vi "Menu Button Facade.vi"(0 "Data In":T4, 2 "Display State In":T2, 3 "Container State":T3) -> (6 "Data Out":T4, 7 "Display State Out":T2, 8 "Action":T1)   [LabVIEW 2011, in "Menu Button Library.lvlib" / "Menu Button xControl.xctl"]
uses:
  Menu Button xControl.xctl
  Menu Button Data.ctl
  <vilib>/_xctls/Container State.ctl
  Menu Button State.ctl
  <vilib>/_xctls/Action.ctl
  <vilib>/_xctls/XControlSupport.lvlib
panel:
  out "Button 0":string
types:
  T1 = typedef "XControlSupport.lvlib/Action.ctl" = cluster{"Data Changed?":bool, "State Changed?":bool, "Action Name":string}
  T2 = typedef "Menu Button Library.lvlib/Menu Button xControl.xctl/Menu Button State.ctl" = cluster{"Number":i32, "Button Text":string, "Background Color":u32}
  T3 = typedef "XControlSupport.lvlib/Container State.ctl" = cluster{"Indicator?":bool, "Run Mode?":bool, " Refnum":refnum<vi>}
  T4 = typedef "Menu Button Library.lvlib/Menu Button xControl.xctl/Menu Button Data.ctl" = bool
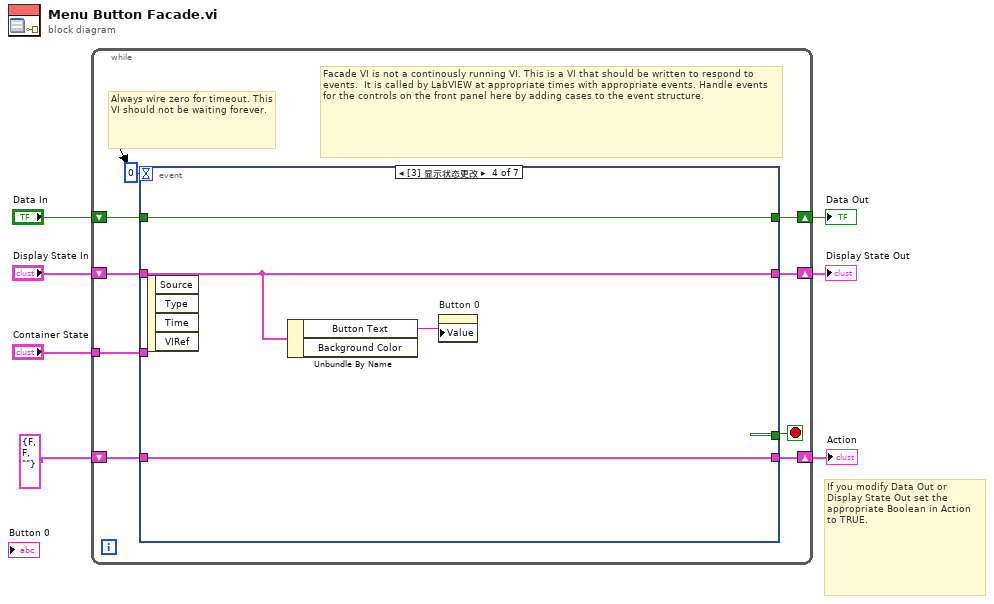
[diagram p0: block diagram]
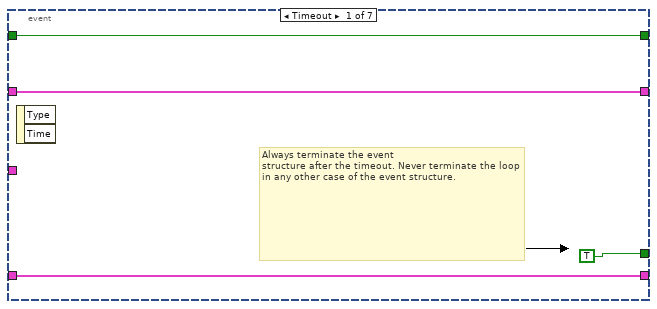
[diagram p2: hidden frame]
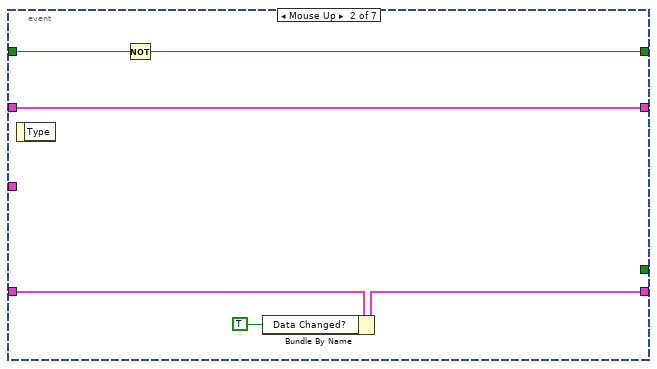
[diagram p3: hidden frame]
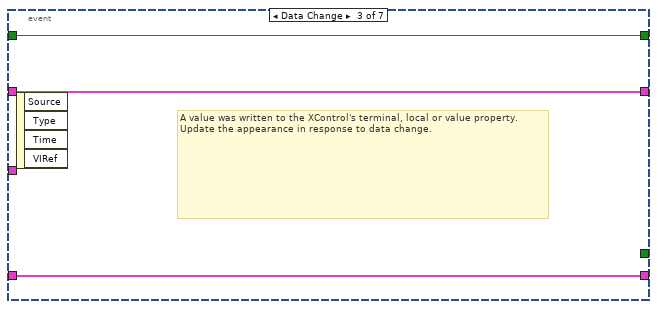
[diagram p4: hidden frame]
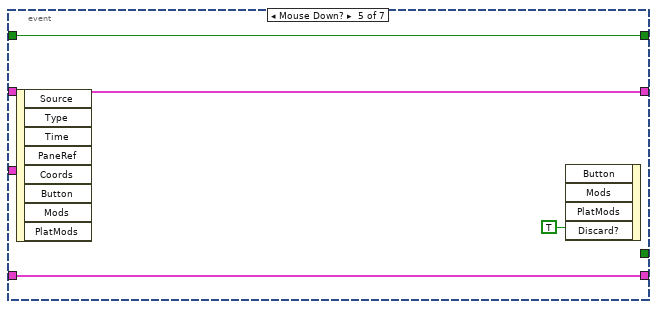
[diagram p5: hidden frame]
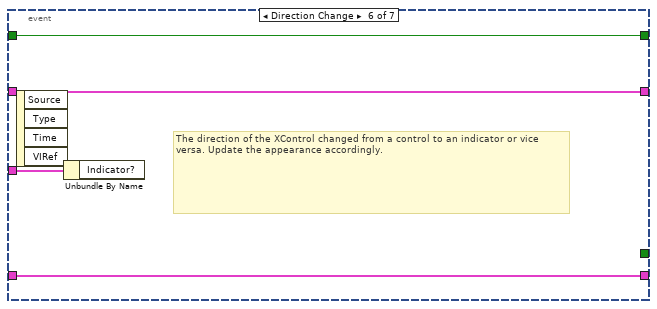
[diagram p6: hidden frame]
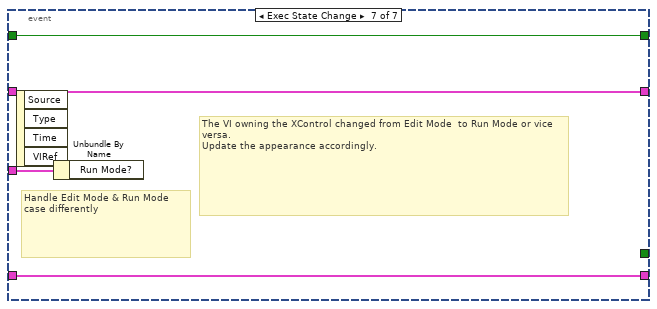
[diagram p7: hidden frame]
diagram:
  # "If you modify Data Out or\nDisplay State Out set the\nappropriate Boolean in Action\nto TRUE."
  n1 = while {
    shift-right: [w15] -> w4
    shift-left: "Display State In" -> [w16]
    tunnel: "Container State" -> [w12]
    shift-right: [w10] -> w7
    shift-left: "Data In" -> [w11]
    shift-right: [w8] -> w2
    shift-left: T1 {"Data Changed?"=FALSE, "State Changed?"=FALSE, "Action Name"=""} ("Action") -> [w9]
    stop <- w14 stop-if-true
    # "Facade VI is not a continously running VI. This is a VI that should be written to respond to events.  It is called by LabVIEW at appropriate times with appropriate events. Handle events for the controls on the front panel here by adding cases to the event structure."
    # "Always wire zero for timeout. This\nVI should not be waiting forever."
    n2 = event shown="[3] 显示状态更改" {
      selector: _ -> [_ _ _ _ _ _ _]
      dyn-events: _ -> [_ _ _ _ _ _ _]
      timeout: 0 -> [_ _ _ _ _ _ _]
      tunnel: w16 -> [w18 w25 w28 w31 w36 w40 w44]
      tunnel: [w18 w25 w28 w31 w36 w40 w44] -> w15
      tunnel: [TRUE _ _ _ _ _ _] -> w14
      tunnel: w12 -> [_ _ _ _ _ w41 w45]
      tunnel: w11 -> [w17 w26 w29 w33 w34 w39 w43]
      tunnel: [w17 w24 w29 w33 w34 w39 w43] -> w10
      tunnel: [w19 w22 w27 w32 w35 w38 w42] -> w8
      tunnel: w9 -> [w19 w23 w27 w32 w35 w38 w42]
      event Timeout {
        # "Always terminate the event\nstructure after the timeout. Never terminate the loop in any other case of the event structure."
        n3 = event-data() -> ()  [unwired: 1 in, 2 out]
      }
      event Mouse Up {
        n4 = event-data() -> ()  [unwired: 1 in, 1 out]
        n5 = Not(x=w26) -> (.not. x?=w24:T4)
        n6 = Bundle By Name(cluster=w23, "Data Changed?"=TRUE) -> (w22:T1)
      }
      event Data Change {
        # "A value was written to the XControl's terminal, local or value property.\nUpdate the appearance in response to data change."
        n7 = event-data() -> ()  [unwired: 1 in, 4 out]
      }
      event Display State Change {
        n8 = event-data() -> ()  [unwired: 1 in, 4 out]
        n9 = Unbundle By Name(w31) -> ("Button Text"=w30:string)  [unwired: 1 out]
        n10 = property on="Button 0" class="Str"("Value"=w30) -> ()  [unwired: 2 in, 2 out]
      }
      event Mouse Down? {
        n11 = event-data() -> ()  [unwired: 1 in, 8 out]
        n12 = event-data("Discard?"=TRUE) -> ()  [unwired: 4 in, 1 out]
      }
      event Direction Change {
        # "The direction of the XControl changed from a control to an indicator or vice versa. Update the appearance accordingly."
        n13 = event-data() -> ()  [unwired: 1 in, 4 out]
        n14 = Unbundle By Name(w41) -> ()  [unwired: 1 out]
      }
      event Exec State Change {
        # "The VI owning the XControl changed from Edit Mode  to Run Mode or vice versa.\nUpdate the appearance accordingly."
        # "Handle Edit Mode & Run Mode\ncase differently"
        n15 = event-data() -> ()  [unwired: 1 in, 4 out]
        n16 = Unbundle By Name(w45) -> ()  [unwired: 1 out]
      }
    }
  }
  "Display State Out" <- w4
  "Data Out" <- w7
  "Action" <- w2
